vi "SetSimOptions.vi"(6 "Legacy (f)?":bool, 8 "error in (no error)":errorcluster, 10 "SIM OPTIONS":T1) -> (0 "error out":errorcluster)   [LabVIEW 2011]
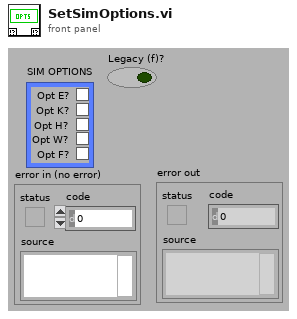
[diagram p1: front panel]
types:
  T1 = cluster{"Opt E?":bool, "Opt K?":bool, "Opt H?":bool, "Opt W?":bool, "Opt F?":bool}
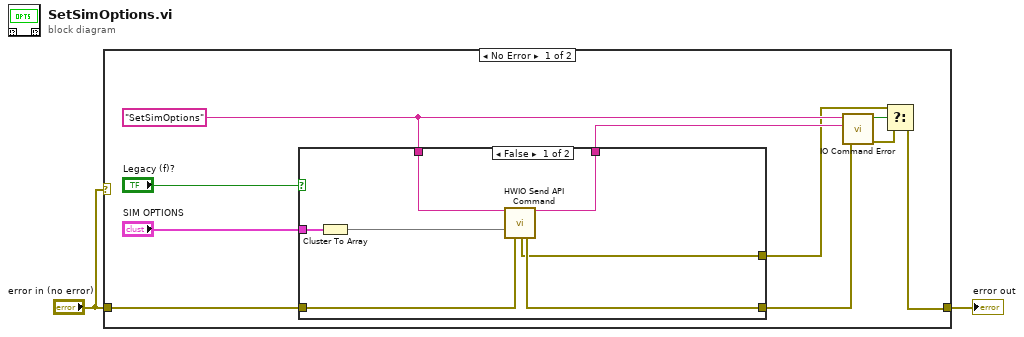
[diagram p0: block diagram]
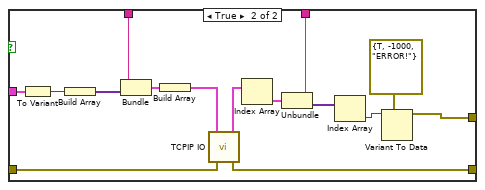
[diagram p2: hidden frame]
diagram:
  n1 = case shown="No Error" "error in (no error)" {
    tunnel: "error in (no error)" -> [w12 w35]
    tunnel: [w5 w35] -> w2
    frame No Error {
      w11 = "SetSimOptions"
      n2 = case shown="False" "Legacy (f)?" {
        tunnel: w12 -> [w19 w32]
        tunnel: w11 -> [w16 w30]
        tunnel: [w18 w29] -> w10
        tunnel: [w17 w25] -> w9
        tunnel: "SIM OPTIONS" -> [w15 w24]
        tunnel: [w13 w20] -> w4
        frame False {
          n3 = Cluster To Array(cluster=w15) -> (array=w14:bool[])
          n4 = call "HWIO Send API Command.vi"("Action"=w16, "Boolean"=w14, "error in (no error)"=w19) -> ("Action out"=w17:string, "HWError"=w13:errorcluster, "error out"=w18:errorcluster)  [unwired: 5 in, 5 out]
        }
        frame True {
          n5 = To Variant(anything=w24) -> (Variant=w34:variant)
          n6 = Build Array(w34) -> (w33:variant[])
          n7 = Bundle(w30, w33) -> (w31:cluster{string, variant[]})  [unwired: 1 out]
          n8 = Build Array(w31) -> (w28:cluster{string, variant[]}[])
          n9 = call "TCPIP IO.vi"("error in (no error)"=w32, "Commands"=w28) -> ("error out"=w29:errorcluster, "Responses"=w27:cluster{string, variant[]}[])  [unwired: 1 in, 3 out]
          n10 = Index Array(array=w27) -> (element=w26:cluster{string, variant[]})  [unwired: 1 in]
          n11 = Unbundle(w26) -> (w25:string, w21:variant[])
          n12 = Index Array(array=w21) -> (element=w23:variant)  [unwired: 1 in]
          n13 = Variant To Data(type=errorcluster {"status"=TRUE, "code"=-1000, "source"="ERROR!"} ("error out"), Variant=w23) -> (data=w20:errorcluster)  [unwired: 1 in, 1 out]
        }
      }
      n14 = call "IO Command Error.vi"("error in (no error)"=w10, "Command Returned (\"\")"=w9, "Command Sent (\"\")"=w11) -> ("error out"=w6:errorcluster, "HW ERR?"=w7:bool)  [unwired: 3 out]
      n15 = Select(t=w4, s=w7, f=w6) -> (s? t:f=w5:errorcluster)
    }
    frame Error {
    }
  }
  "error out" <- w2
